vi "Path To Command Line String.vi"(1 "path":path) -> (0 "string":string)   [LabVIEW 2017]
doc: "Converts <B>path</B> into a <B>string</B> describing a path in the standard format for the command line of the platform."
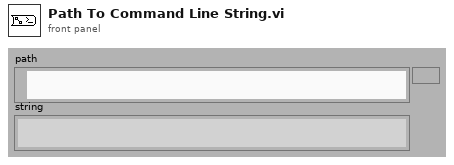
[diagram p1: front panel]
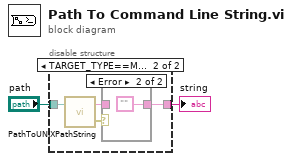
[diagram p0: block diagram]
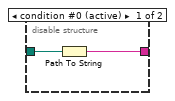
[diagram p2: hidden frame]
diagram:
  n1 = disable-structure shown="TARGET_TYPE==Mac&&TARGET_BITNESS!=64" {
    disable-tunnel: "path" -> [w4 w8]
    disable-tunnel: [w3 w5] -> w1
    frame condition #0 (active) {
      n2 = Path To String(path=w4) -> (string=w3:string)
    }
    frame condition #1 {
      n3 = call <vilib>:"PathToUNIXPathString.vi"("LV Path"=w8) -> ("error out"=w7:errorcluster, "UNIX Path"=w6:string)  [unwired: 1 in]
      n4 = case shown="Error" w7 {
        tunnel: w6 -> [w9 _]
        tunnel: [w9 ""] -> w5
        frame No Error {
        }
        frame Error {
        }
      }
    }
  }
  "string" <- w1
